vi "about Open Connection DriverConnect.vi"(5 "error in (no error)":errorcluster, 8 "ODBC Database (\"\")":path) -> (0 "error out":errorcluster, 3 "Connection Refnum":T1)   [LabVIEW 2011]
doc: "Réalise l'ensemble des étapes nécéssaires à la mise en place de la connection avec la base de données. Etablit le cas échéant l'utilisation des transactions."
uses:
  Summitek EXT/ODBC/SQL Controls/Connection Refnum.ctl
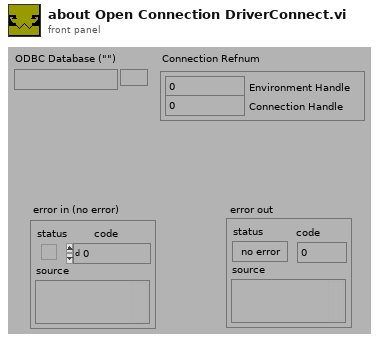
[diagram p1: front panel]
types:
  T1 = typedef "Connection Refnum.ctl" = cluster{"Environment Handle":i32, "Connection Handle":i32}
  T2 = cluster{"Environment Handle":i32, "Connection Handle":i32}
  T3 = enum16{"NOPE", "SQL_HANDLE_ENV", "SQL_HANDLE_DBC", "SQL_HANDLE_STMT", "SQL_HANDLE_DESC"}
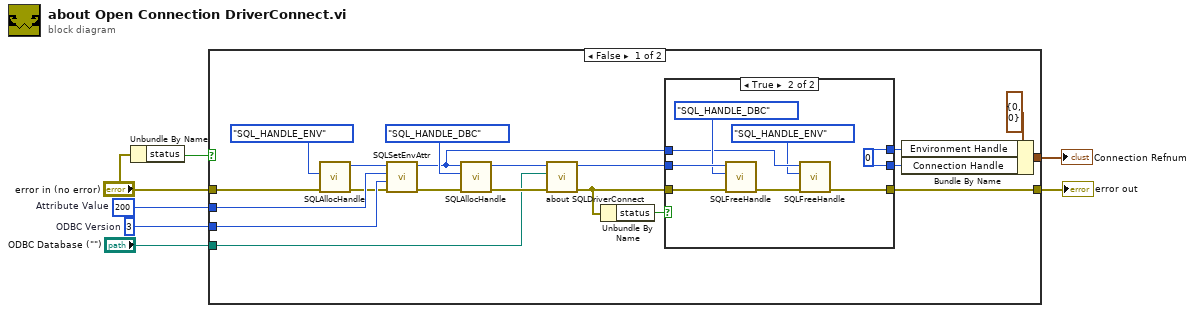
[diagram p0: block diagram]
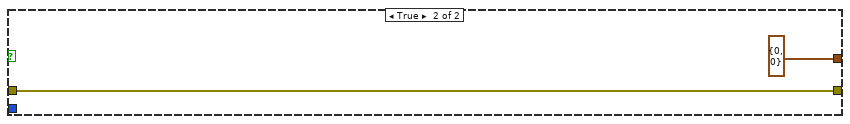
[diagram p3: hidden frame]
diagram:
  w5 = u32 3  # ODBC Version
  w6 = 200  # Attribute Value
  n1 = Unbundle By Name("error in (no error)") -> ("status"=w1:bool)
  n2 = case shown="False" w1 {
    tunnel: "ODBC Database (\"\")" -> [w8 _]
    tunnel: w6 -> [w24 _]
    tunnel: w5 -> [w23 _]
    tunnel: [w20 T2 {"Environment Handle"=0, "Connection Handle"=0} ("Connection Refnum")] -> w4
    tunnel: [w14 w40] -> w3
    tunnel: "error in (no error)" -> [w13 w40]
    frame False {
      n3 = call "SQLAllocHandle.vi"("error in (no error)"=w13, "HandleType"=T3."SQL_HANDLE_ENV") -> ("error out"=w17:errorcluster, "OutputHandle"=w22:i32)  [unwired: 1 in, 3 out]
      n4 = call "SQLSetEnvAttr.vi"("error in (no error)"=w17, "AttributeValue"=w23, "AttributePosition"=w24, "InputHandle"=w22) -> ("error out"=w16:errorcluster, "OutputHandle"=w25:i32)  [unwired: 2 out]
      n5 = call "SQLAllocHandle.vi"("error in (no error)"=w16, "HandleType"=T3."SQL_HANDLE_DBC", "InputHandle"=w25) -> ("error out"=w10:errorcluster, "OutputHandle"=w12:i32)  [unwired: 3 out]
      n6 = call "about SQLDriverConnect.vi"("error in (no error)"=w10, "Database Path (empty)"=w8, "InputHandle"=w12) -> ("error out"=w9:errorcluster, "OutputHandle"=w11:i32)  [unwired: 4 out]
      n7 = Unbundle By Name(w9) -> ("status"=w15:bool)
      n8 = case shown="True" w15 {
        tunnel: w11 -> [w29 w38]
        tunnel: w25 -> [w30 w34]
        tunnel: [w30 w37] -> w19
        tunnel: [w29 w37] -> w18
        tunnel: [w28 w32] -> w14
        tunnel: w9 -> [w28 w31]
        frame False {
        }
        frame True {
          w37 = 0 ("OutputHandle")
          n9 = call "SQLFreeHandle.vi"("error in (no error)"=w31, "HandleType"=T3."SQL_HANDLE_DBC", "InputHandle"=w38) -> ("error out"=w35:errorcluster)  [unwired: 4 out]
          n10 = call "SQLFreeHandle.vi"("error in (no error)"=w35, "HandleType"=T3."SQL_HANDLE_ENV", "InputHandle"=w34) -> ("error out"=w32:errorcluster)  [unwired: 4 out]
        }
      }
      n11 = Bundle By Name(cluster=T2 {"Environment Handle"=0, "Connection Handle"=0} ("Connection Refnum"), "Environment Handle"=w19, "Connection Handle"=w18) -> (w20:T2)
    }
    frame True {
    }
  }
  "Connection Refnum" <- w4
  "error out" <- w3
